vi "AlliGator Get Available Fitting Parameters.vi"(11 "Parameter Names":T1[](array[typedef])) -> (3 "Missing Parameter Names":T1[](array[typedef]))   [LabVIEW 2021, in "AlliGator Settings.lvlib"]
doc: "Returns list of parameters not in the <B>Parameter Names</B> list."
uses:
  Fits/IRF(X)PSED/Decay Fit Parameters In List.ctl
  325204a7-54f9-4925-b933-958484244497.vi
  <userlib>/_OpenG.lib/array/array.llb/Filter 1D Array (I32)__ogtk.vi
  AlliGator Settings.lvlib
  <userlib>/_OpenG.lib/array/array.llb/openg_array.lvlib
  Fits/Fits.lvlib
panel:
  in  "Fit Parameter used to access parameter name list":T1
  # "see the AlliGator License on the block diagram (Ctrl+E or Window:Show Block Diagram)"
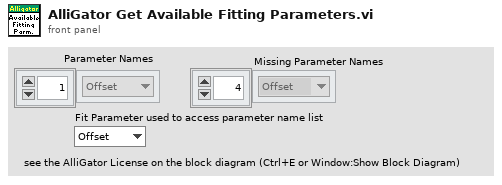
[diagram p1: front panel]
types:
  T1 = typedef "Fits.lvlib/Decay Fit Parameters In List.ctl" = enum16{"Offset", "Baseline", "A_1", "tau_1", "A_2", "tau_2"}
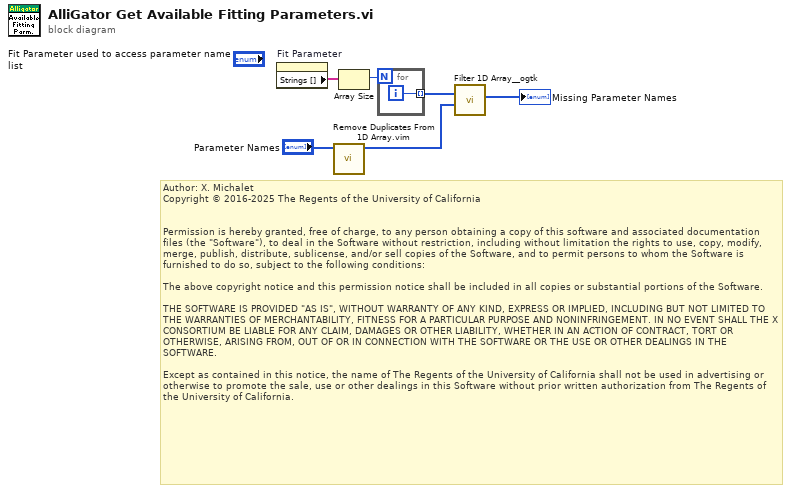
[diagram p0: block diagram]
diagram:
  # "Author: X. Michalet\nCopyright © 2016-2025 The Regents of the University of California\n \n\nPermission is hereby granted, free of charge, to any person obtaining a copy of this software and associated documentation files (the \"Software\"), to deal in the Software without restriction, including without limitation the rights to use, copy, modify, merge, publish, distribute, sublicense, and/or sell copies of the Software, and to permit persons to whom the Software is furnished to do so, subject to the following conditions:\n\nThe above copyright notice and this permission notice shall be included in all copies or substantial portions of the Software.\n\nTHE SOFTWARE IS PROVIDED \"AS IS\", WITHOUT WARRANTY OF ANY KIND, EXPRESS OR IMPLIED, INCLUDING BUT NOT LIMITED TO THE WARRANTIES OF MERCHANTABILITY, FITNESS FOR A PARTICULAR PURPOSE AND NONINFRINGEMENT. IN NO EVENT SHALL THE X CONSORTIUM BE LIABLE FOR ANY CLAIM, DAMAGES OR OTHER LIABILITY, WHETHER IN AN ACTION OF CONTRACT, TORT OR OTHERWISE, ARISING FROM, OUT OF OR IN CONNECTION WITH THE SOFTWARE OR THE USE OR OTHER DEALINGS IN THE SOFTWARE.\n\nExcept as contained in this notice, the name of The Regents of the University of California shall not be used in advertising or otherwise to promote the sale, use or other dealings in this Software without prior written authorization from The Regents of the University of California."
  n1 = property on="Fit Parameter" class="Enum (strict)"() -> ("Strings []"=w5:string[])  [unwired: 2 in, 2 out]
  n2 = call "Remove Duplicates From 1D Array.vim"("array"="Parameter Names") -> ("array with duplicates removed"=w2:T1[])  [unwired: 10 in]
  n3 = Array Size(array=w5) -> (size(s)=w4:i32)
  n4 = for {
    N: w4 -> [_]
    tunnel: [w7] -> w3 mode=indexing
    i -> [w7]
  }
  n5 = call-poly <userlib>:"Filter 1D Array__ogtk.vi"("items to filter"=w2, "array"=w3) -> ("filtered array"=→"Missing Parameter Names":i32[])  [unwired: 4 in, 1 out]
